vi "TabToDict.vi"(9 "String Value":string[](array[string]), 10 "Int Value":i32[](array[numeric]), 11 "String key":string[](array[string])) -> (2 "Dict with string value":string, 3 "Dict with int value":string)   [LabVIEW 2020]
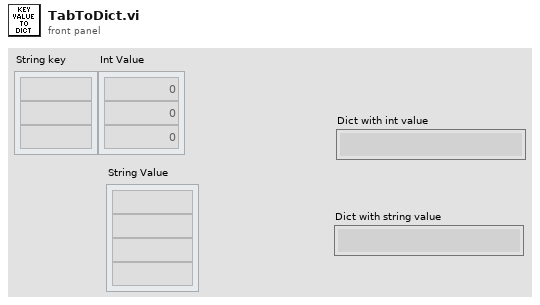
[diagram p1: front panel]
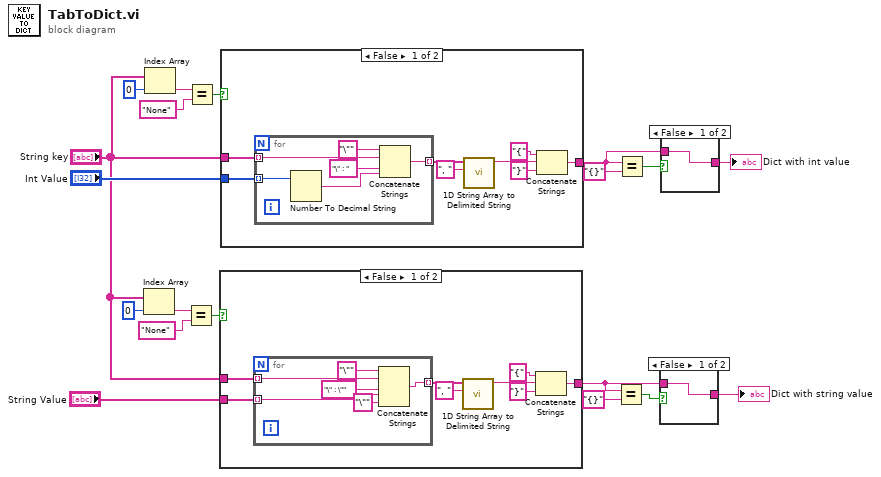
[diagram p0: block diagram]
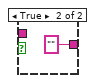
[diagram p2: hidden frame]
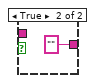
[diagram p3: hidden frame]
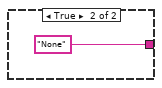
[diagram p4: hidden frame]
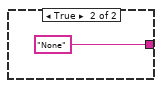
[diagram p5: hidden frame]
diagram:
  n1 = Index Array(array="String key", index=0 ("indice")) -> (element=w12:string)
  n2 = Index Array(array="String key", index=0 ("indice")) -> (element=w17:string)
  n3 = Equal?(x=w12, y="None") -> (x = y?=w10:bool)
  n4 = Equal?(x=w17, y="None") -> (x = y?=w15:bool)
  n5 = case shown="False" w10 {
    tunnel: "String key" -> [w27 _]
    tunnel: "String Value" -> [w26 _]
    tunnel: [w20 "None"] -> w2
    frame False {
      n6 = for {
        tunnel: w27 -> [w33] mode=indexing
        tunnel: w26 -> [w29] mode=indexing
        tunnel: [w30] -> w25 mode=indexing
        n7 = Concatenate Strings("\"" ("chaîne"), w33, "\" : \"" ("chaîne"), w29, "\"" ("string")) -> (w30:string)
      }
      n8 = call <vilib>:"1D String Array to Delimited String.vi"("delimiter"=", ", "string array"=w25) -> ("delimited string"=w23:string)  [unwired: 9 in]
      n9 = Concatenate Strings("{", w23, "}" ("chaîne")) -> (w20:string)
    }
    frame True {
    }
  }
  n10 = case shown="False" w15 {
    tunnel: "String key" -> [w42 _]
    tunnel: "Int Value" -> [w41 _]
    tunnel: [w35 "None"] -> w5
    frame False {
      n11 = for {
        tunnel: w42 -> [w48] mode=indexing
        tunnel: w41 -> [w45] mode=indexing
        tunnel: [w43] -> w40 mode=indexing
        n12 = Number To Decimal String(number=w45) -> (decimal integer string=w44:string)  [unwired: 1 in]
        n13 = Concatenate Strings("\"" ("chaîne"), w48, "\" : " ("chaîne"), w44) -> (w43:string)
      }
      n14 = call <vilib>:"1D String Array to Delimited String.vi"("delimiter"=", ", "string array"=w40) -> ("delimited string"=w38:string)  [unwired: 9 in]
      n15 = Concatenate Strings("{", w38, "}" ("chaîne")) -> (w35:string)
    }
    frame True {
    }
  }
  n16 = Equal?(x=w2, y="{}") -> (x = y?=w3:bool)
  n17 = Equal?(x=w5, y="{}") -> (x = y?=w7:bool)
  n18 = case shown="False" w3 {
    tunnel: [w50 ""] -> w1
    tunnel: w2 -> [w50 _]
    frame False {
    }
    frame True {
    }
  }
  "Dict with string value" <- w1
  n19 = case shown="False" w7 {
    tunnel: [w52 ""] -> w6
    tunnel: w5 -> [w52 _]
    frame False {
    }
    frame True {
    }
  }
  "Dict with int value" <- w6
